vi "_PC_Pub openHelperHtml.vi"(2 "error in (no error)":errorcluster, 3 "procType":enum16{"none", "MSProcess", "SignalProcess"}(ring)) -> (0 "error out":errorcluster, 1 "URL out":string)   [LabVIEW 2018]
uses:
  <vilib>/Platform/browser.llb/Open URL in Default Browser (path).vi
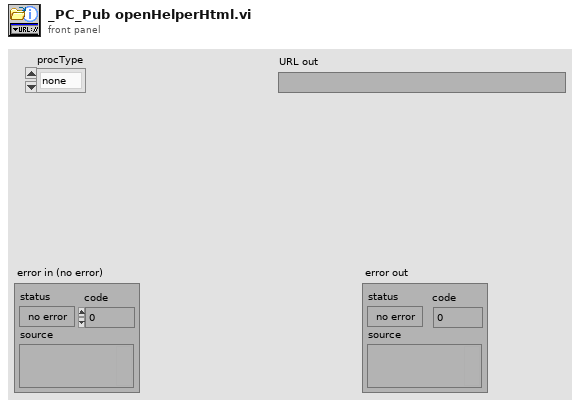
[diagram p1: front panel]
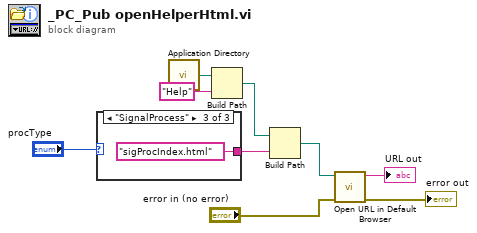
[diagram p0: block diagram]
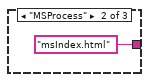
[diagram p3: hidden frame]
diagram:
  n1 = case shown="\"SignalProcess\"" "procType" {
    tunnel: [_ "msIndex.html" ("name or relative path") "sigProcIndex.html" ("name or relative path")] -> w1
    frame "none", Default {
    }
    frame "MSProcess" {
    }
    frame "SignalProcess" {
    }
  }
  n2 = call <vilib>:"Application Directory.vi"() -> ("Application Directory"=w9:path)
  n3 = Build Path(base path=w9, name or relative path="Help") -> (appended path=w7:path)
  n4 = Build Path(base path=w7, name or relative path=w1) -> (appended path=w6:path)
  n5 = call-poly <vilib>:"Open URL in Default Browser.vi"("error in (no error)"="error in (no error)", "path"=w6) -> ("error out"=→"error out":errorcluster, "URL out"=→"URL out":string)  [unwired: 4 in]
